vi "DataMerger.vi"() -> ()   [LabVIEW 2011]
panel:
  in  "R_BlobLinePairing":T1(array[cluster])
  in  "L_BlobLinePairing":T1(array[cluster])
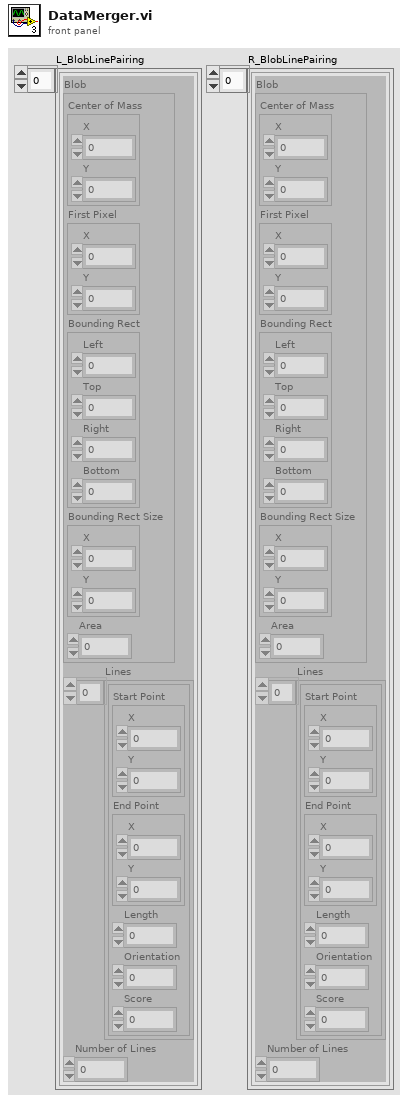
[diagram p1: front panel]
types:
  T1 = cluster{"Blob":cluster{"Center of Mass":cluster{"X":dbl, "Y":dbl}, "First Pixel":cluster{"X":dbl, "Y":dbl}, "Bounding Rect":cluster{"Left":dbl, "Top":dbl, "Right":dbl, "Bottom":dbl}, "Bounding Rect Size":cluster{"X":dbl, "Y":dbl}, "Area":dbl}, "Lines":cluster{"Start Point":cluster{"X":sgl, "Y":sgl}, "End Point":cluster{"X":sgl, "Y":sgl}, "Length":dbl, "Orientation":dbl, "Score":dbl}[], "Number of Lines":i32}[]
  T2 = cluster{cluster{"BlobData In[0]":dbl, "BlobData In[1]":dbl}, cluster{"BlobData In[2]":dbl, "BlobData In[3]":dbl}, cluster{"BlobData In[4]":dbl, "BlobData In[5]":dbl, "BlobData In[6]":dbl, "BlobData In[7]":dbl}, cluster{"BlobData In[8]":dbl, "BlobData In[9]":dbl}, "BlobData In[10]":dbl}
  T3 = cluster{"Center of Mass":cluster{"X":dbl, "Y":dbl}, "First Pixel":cluster{"X":dbl, "Y":dbl}, "Bounding Rect":cluster{"Left":dbl, "Top":dbl, "Right":dbl, "Bottom":dbl}, "Bounding Rect Size":cluster{"X":dbl, "Y":dbl}, "Area":dbl}
  T4 = cluster{"Left":dbl, "Top":dbl, "Right":dbl, "Bottom":dbl}
  T5 = cluster{"Center of Mass":cluster{"BlobData In[0]":dbl, "BlobData In[1]":dbl}, "First Pixel":cluster{"BlobData In[2]":dbl, "BlobData In[3]":dbl}, "Bounding Rect":cluster{"BlobData In[4]":dbl, "BlobData In[5]":dbl, "BlobData In[6]":dbl, "BlobData In[7]":dbl}, "Bounding Rect Size":cluster{"BlobData In[8]":dbl, "BlobData In[9]":dbl}, "BlobData In[10]":dbl}
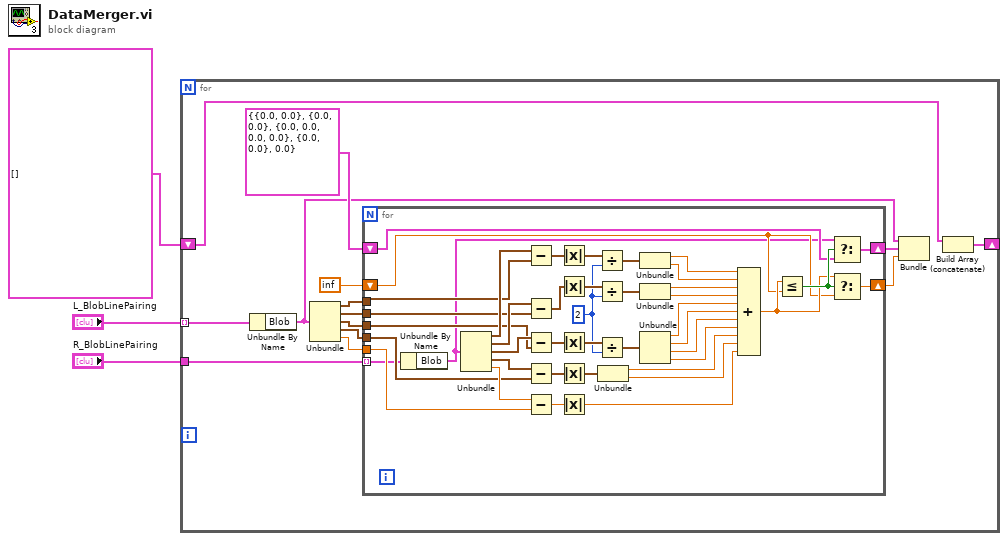
[diagram p0: block diagram]
diagram:
  n1 = for {
    tunnel: "L_BlobLinePairing" -> [w5] mode=indexing
    tunnel: "R_BlobLinePairing" -> [w17]
    shift-right: [w12] -> _
    shift-left: T1 [] ("R_BlobLinePairing") -> [w11]
    n2 = Unbundle By Name(w5) -> ("Blob"=w4:T3)
    n3 = Unbundle(w4) -> ("Center of Mass"=w10:cluster{"X":dbl, "Y":dbl}, "First Pixel"=w9:cluster{"X":dbl, "Y":dbl}, "Bounding Rect"=w8:T4, "Bounding Rect Size"=w16:cluster{"X":dbl, "Y":dbl}, "Area"=w15:dbl)
    n4 = for {
      tunnel: w17 -> [w19] mode=indexing
      tunnel: w15 -> [w57]
      tunnel: w16 -> [w55]
      shift-right: [w24] -> w13
      shift-left: T2 {{"BlobData In[0]"=0.0, "BlobData In[1]"=0.0}, {"BlobData In[2]"=0.0, "BlobData In[3]"=0.0}, {"BlobData In[4]"=0.0, "BlobData In[5]"=0.0, "BlobData In[6]"=0.0, "BlobData In[7]"=0.0}, {"BlobData In[8]"=0.0, "BlobData In[9]"=0.0}, "BlobData In[10]"=0.0} -> [w28]
      tunnel: w10 -> [w50]
      tunnel: w9 -> [w49]
      tunnel: w8 -> [w48]
      shift-right: [w25] -> w6
      shift-left: inf -> [w26]
      w20 = 2
      n5 = Unbundle By Name(w19) -> ("Blob"=w18:T3)
      n6 = Unbundle(w18) -> ("Center of Mass"=w53:cluster{"X":dbl, "Y":dbl}, "First Pixel"=w52:cluster{"X":dbl, "Y":dbl}, "Bounding Rect"=w51:T4, "Bounding Rect Size"=w59:cluster{"X":dbl, "Y":dbl}, "Area"=w58:dbl)
      n7 = Subtract(x=w53, y=w50) -> (x-y=w47:cluster{"X":dbl, "Y":dbl})
      n8 = Subtract(x=w52, y=w49) -> (x-y=w46:cluster{"X":dbl, "Y":dbl})
      n9 = Subtract(x=w51, y=w48) -> (x-y=w45:T4)
      n10 = Subtract(x=w59, y=w55) -> (x-y=w56:cluster{"X":dbl, "Y":dbl})
      n11 = Subtract(x=w58, y=w57) -> (x-y=w54:dbl)
      n12 = Absolute Value(x=w47) -> (abs(x)=w44:cluster{"X":dbl, "Y":dbl})
      n13 = Absolute Value(x=w46) -> (abs(x)=w43:cluster{"X":dbl, "Y":dbl})
      n14 = Absolute Value(x=w45) -> (abs(x)=w42:T4)
      n15 = Absolute Value(x=w56) -> (abs(x)=w33:cluster{"X":dbl, "Y":dbl})
      n16 = Absolute Value(x=w54) -> (abs(x)=w30:dbl)
      n17 = Divide(x=w44, y=w20) -> (x/y=w23:cluster{"X":dbl, "Y":dbl})
      n18 = Divide(x=w43, y=w20) -> (x/y=w22:cluster{"X":dbl, "Y":dbl})
      n19 = Divide(x=w42, y=w20) -> (x/y=w21:T4)
      n20 = Unbundle(w33) -> ("X"=w32:dbl, "Y"=w31:dbl)
      n21 = Unbundle(w23) -> ("X"=w41:dbl, "Y"=w40:dbl)
      n22 = Unbundle(w22) -> ("X"=w39:dbl, "Y"=w38:dbl)
      n23 = Unbundle(w21) -> ("Left"=w37:dbl, "Top"=w36:dbl, "Right"=w35:dbl, "Bottom"=w34:dbl)
      n24 = Compound Arithmetic op=ADD(w41, w40, w39, w38, w37, w36, w35, w34, w32, w31, w30) -> (w27:dbl)
      n25 = Less Or Equal?(x=w27, y=w26) -> (x <= y?=w29:bool)
      n26 = Select(t=w18, s=w29, f=w28) -> (s? t:f=w24:T5)
      n27 = Select(t=w27, s=w29, f=w26) -> (s? t:f=w25:dbl)
    }
    n28 = Bundle("Blob"=w4, w13, w6) -> ()  [unwired: 1 in, 1 out]
    n29 = Build Array (concatenate)(w11) -> (w12:T1)  [unwired: 1 in]
  }
